vi "main.vi"() -> ()   [LabVIEW 2023] (continued)
  00000004    8        68\t00\t97\tCC\t00\t16\t39\tB4\r\n      3082  1FFFFFFF   00000004    8        00\t20\tFF\tFF\tFF\tFF\tFF\tFF\r\n      3072  1FFFFFFF   00000004    8        00\t20\tFF\tFF\tFF\tFF\tFF\tFF\r\n      3123  0CF101A7   00000004    8        68\t00\t97\tCC\t00\t16\t39\tB6\r\n      3122  1FFFFFFF   00000004    8        00\t00\tFF\tFF\tFF\tFF\tFF\tFF\r\n      3112  1FFFFFFF   00000004    8        00\t20\tFF\tFF\tFF\tFF\tFF\tFF\r\n      3103  0CF102A7   00000004    8        30\t75\tE0\t2E\t80\tFF\tFF\tFD\r\n      3103  0CF101A7   00000004    8        68\t00\t97\tCC\t00\t16\t39\tB5\r\n      3102  1FFFFFFF   00000004    8        00\t00\tFF\tFF\tFF\tFF\tFF\tFF\r\n      3093  18F106A7   00000004    8        00\tF7\tFF\tFF\tFF\tFF\tFF\tAE\r\n      3092  1FFFFFFF   00000004    8        00\t20\tFF\tFF\tFF\tFF\tFF\tFF\r\n      3083  0CF102A7   00000004    8        30\t75\tE0\t2E\t80\tFF\tFF\tFD\r\n      3083  0CF101A7   00000004    8        68\t00\t97\tCC\t00\t16\t39\tB4\r\n      3082  1FFFFFFF   00000004    8        00\t20\tFF\tFF\tFF\tFF\tFF\tFF\r\n      3123  0CF102A7   00000004    8        30\t75\tE0\t2E\t80\tFF\tFF\tFD\r\n      3123  0CF101A7   00000004    8        68\t00\t97\tCC\t00\t16\t39\tB6\r\n      3122  1FFFFFFF   00000004    8        00\t00\tFF\tFF\tFF\tFF\tFF\tFF\r\n      3112  1FFFFFFF   00000004    8        00\t20\tFF\tFF\tFF\tFF\tFF\tFF\r\n      3103  0CF102A7   00000004    8        30\t75\tE0\t2E\t80\tFF\tFF\tFD\r\n      3103  0CF101A7   00000004    8        68\t00\t97\tCC\t00\t16\t39\tB5\r\n      3102  1FFFFFFF   00000004    8        00\t00\tFF\tFF\tFF\tFF\tFF\tFF\r\n      3093  18F106A7   00000004    8        00\tF7\tFF\tFF\tFF\tFF\tFF\tAE\r\n      3092  1FFFFFFF   00000004    8        00\t20\tFF\tFF\tFF\tFF\tFF\tFF\r\n      3083  0CF102A7   00000004    8        30\t75\tE0\t2E\t80\tFF\tFF\tFD\r\n      3083  0CF101A7   00000004    8        68\t00\t97\tCC\t00\t16\t39\tB4\r\n      3132  1FFFFFFF   00000004    8        00\t20\tFF\tFF\tFF\tFF\tFF\tFF\r\n      3123  0CF102A7   00000004    8        30\t75\tE0\t2E\t80\tFF\tFF\tFD\r\n      3123  0CF101A7   00000004    8        68\t00\t97\tCC\t00\t16\t39\tB6\r\n      3122  1FFFFFFF   00000004    8        00\t00\tFF\tFF\tFF\tFF\tFF\tFF\r\n      3112  1FFFFFFF   00000004    8        00\t20\tFF\tFF\tFF\tFF\tFF\tFF\r\n      3103  0CF102A7   00000004    8        30\t75\tE0\t2E\t80\tFF\tFF\tFD\r\n      3103  0CF101A7   00000004    8        68\t00\t97\tCC\t00\t16\t39\tB5\r\n      3102  1FFFFFFF   00000004    8        00\t00\tFF\tFF\tFF\tFF\tFF\tFF\r\n      3093  18F106A7   00000004    8        00\tF7\tFF\tFF\tFF\tFF\tFF\tAE\r\n      3092  1FFFFFFF   00000004    8        00\t20\tFF\tFF\tFF\tFF\tFF\tFF\r\n      3083  0CF102A7   00000004    8        30\t75\tE0\t2E\t80\tFF\tFF\tFD\r\n      3141  18F11FF0   00000004    8        FF\t3F\t90\t68\t88\t1B\t10\t7C\r\n      3132  1FFFFFFF   00000004    8        00\t20\tFF\tFF\tFF\tFF\tFF\tFF\r\n      3123  0CF102A7   00000004    8        30\t75\tE0\t2E\t80\tFF\tFF\tFD\r\n      3123  0CF101A7   00000004    8        68\t00\t97\tCC\t00\t16\t39\tB6\r\n      3122  1FFFFFFF   00000004    8        00\t00\tFF\tFF\tFF\tFF\tFF\tFF\r\n      3112  1FFFFFFF   00000004    8        00\t20\tFF\tFF\tFF\tFF\tFF\tFF\r\n      3103  0CF102A7   00000004    8        30\t75\tE0\t2E\t80\tFF\tFF\tFD\r\n      3103  0CF101A7   00000004    8        68\t00\t97\tCC\t00\t16\t39\tB5\r\n      3102  1FFFFFFF   00000004    8        00\t00\tFF\tFF\tFF\tFF\tFF\tFF\r\n      3093  18F106A7   00000004    8        00\tF7\tFF\tFF\tFF\tFF\tFF\tAE\r\n      3092  1FFFFFFF   00000004    8        00\t20\tFF\tFF\tFF\tFF\tFF\tFF\r\n      3142  18F120F0   00000004    8        2B\t75\t60\tB1\tB0\t01\tFF\tFF\r\n      3141  18F11FF0   00000004    8        FF\t3F\t90\t68\t88\t1B\t10\t7C\r\n      3132  1FFFFFFF   00000004    8        00\t20\tFF\tFF\tFF\tFF\tFF\tFF\r\n      3123  0CF102A7   00000004    8        30\t75\tE0\t2E\t80\tFF\tFF\tFD\r\n      3123  0CF101A7   00000004    8        68\t00\t97\tCC\t00\t16\t39\tB6\r\n      3122  1FFFFFFF   00000004    8        00\t00\tFF\tFF\tFF\tFF\tFF\tFF\r\n      3112  1FFFFFFF   00000004    8        00\t20\tFF\tFF\tFF\tFF\tFF\tFF\r\n      3103  0CF102A7   00000004    8        30\t75\tE0\t2E\t80\tFF\tFF\tFD\r\n      3103  0CF101A7   00000004    8        68\t00\t97\tCC\t00\t16\t39\tB5\r\n      3102  1FFFFFFF   00000004    8        00\t00\tFF\tFF\tFF\tFF\tFF\tFF\r\n      3093  18F106A7   00000004    8        00\tF7\tFF\tFF\tFF\tFF\tFF\tAE\r\n      3143  0CF101A7   00000004    8        68\t00\t97\tCC\t00\t16\t39\tB7\r\n      3142  18F120F0   00000004    8        2B\t75\t60\tB1\tB0\t01\tFF\tFF\r\n      3141  18F11FF0   00000004    8        FF\t3F\t90\t68\t88\t1B\t10\t7C\r\n      3132  1FFFFFFF   00000004    8        00\t20\tFF\tFF\tFF\tFF\tFF\tFF\r\n      3123  0CF102A7   00000004    8        30\t75\tE0\t2E\t80\tFF\tFF\tFD\r\n      3123  0CF101A7   00000004    8        68\t00\t97\tCC\t00\t16\t39\tB6\r\n      3122  1FFFFFFF   00000004    8        00\t00\tFF\tFF\tFF\tFF\tFF\tFF\r\n      3112  1FFFFFFF   00000004    8        00\t20\tFF\tFF\tFF\tFF\tFF\tFF\r\n      3103  0CF102A7   00000004    8        30\t75\tE0\t2E\t80\tFF\tFF\tFD\r\n      3103  0CF101A7   00000004    8        68\t00\t97\tCC\t00\t16\t39\tB5\r\n      3102  1FFFFFFF   00000004    8        00\t00\tFF\tFF\tFF\tFF\tFF\tFF\r\n      3143  0CF102A7   00000004    8        30\t75\tE0\t2E\t80\tFF\tFF\tFD\r\n      3143  0CF101A7   00000004    8        68\t00\t97\tCC\t00\t16\t39\tB7\r\n      3142  18F120F0   00000004    8        2B\t75\t60\tB1\tB0\t01\tFF\tFF\r\n      3141  18F11FF0   00000004    8        FF\t3F\t90\t68\t88\t1B\t10\t7C\r\n      3132  1FFFFFFF   00000004    8        00\t20\tFF\tFF\tFF\tFF\tFF\tFF\r\n      3123  0CF102A7   00000004    8        30\t75\tE0\t2E\t80\tFF\tFF\tFD\r\n      3123  0CF101A7   00000004    8        68\t00\t97\tCC\t00\t16\t39\tB6\r\n      3122  1FFFFFFF   00000004    8        00\t00\tFF\tFF\tFF\tFF\tFF\tFF\r\n      3112  1FFFFFFF   00000004    8        00\t20\tFF\tFF\tFF\tFF\tFF\tFF\r\n      3103  0CF102A7   00000004    8        30\t75\tE0\t2E\t80\tFF\tFF\tFD\r\n      3103  0CF101A7   00000004    8        68\t00\t97\tCC\t00\t16\t39\tB5\r\n      3144  0C3C4D4A   00000004    8        BE\tFF\tFF\t7F\t18\tFF\tFF\t57\r\n      3143  0CF102A7   00000004    8        30\t75\tE0\t2E\t80\tFF\tFF\tFD\r\n      3143  0CF101A7   00000004    8        68\t00\t97\tCC\t00\t16\t39\tB7\r\n      3142  18F120F0   00000004    8        2B\t75\t60\tB1\tB0\t01\tFF\tFF\r\n      3141  18F11FF0   00000004    8        FF\t3F\t90\t68\t88\t1B\t10\t7C\r\n      3132  1FFFFFFF   00000004    8        00\t20\tFF\tFF\tFF\tFF\tFF\tFF\r\n      3123  0CF102A7   00000004    8        30\t75\tE0\t2E\t80\tFF\tFF\tFD\r\n      3123  0CF101A7   00000004    8        68\t00\t97\tCC\t00\t16\t39\tB6\r\n      3122  1FFFFFFF   00000004    8        00\t00\tFF\tFF\tFF\tFF\tFF\tFF\r\n      3112  1FFFFFFF   00000004    8        00\t20\tFF\tFF\tFF\tFF\tFF\tFF\r\n      3103  0CF102A7   00000004    8        30\t75\tE0\t2E\t80\tFF\tFF\tFD\r\n      3144  0CF103A7   00000004    8        17\t1F\t08\t60\tB1\t1F\t08\t57\r\n      3144  0C3C4D4A   00000004    8        BE\tFF\tFF\t7F\t18\tFF\tFF\t57\r\n      3143  0CF102A7   00000004    8        30\t75\tE0\t2E\t80\tFF\tFF\tFD\r\n      3143  0CF101A7   00000004    8        68\t00\t97\tCC\t00\t16\t39\tB7\r\n      3142  18F120F0   00000004    8        2B\t75\t60\tB1\tB0\t01\tFF\tFF\r\n      3141  18F11FF0   00000004    8        FF\t3F\t90\t68\t88\t1B\t10\t7C\r\n      3132  1FFFFFFF   00000004    8        00\t20\tFF\tFF\tFF\tFF\tFF\tFF\r\n      3123  0CF102A7   00000004    8        30\t75\tE0\t2E\t80\tFF\tFF\tFD\r\n      3123  0CF101A7   00000004    8        68\t00\t97\tCC\t00\t16\t39\tB6\r\n      3122  1FFFFFFF   00000004    8        00\t00\tFF\tFF\tFF\tFF\tFF\tFF\r\n      3112  1FFFFFFF   00000004    8        00\t20\tFF\tFF\tFF\tFF\tFF\tFF\r\n      3145  0CF104A7   00000004    8        F0\t60\t22\tFC\tFF\tFF\tFF\t57\r\n      3144  0CF103A7   00000004    8        17\t1F\t08\t60\tB1\t1F\t08\t57\r\n      3144  0C3C4D4A   00000004    8        BE\tFF\tFF\t7F\t18\tFF\tFF\t57\r\n      3143  0CF102A7   00000004    8        30\t75\tE0\t2E\t80\tFF\tFF\tFD\r\n      3143  0CF101A7   00000004    8        68\t00\t97\tCC\t00\t16\t39\tB7\r\n      3142  18F120F0   00000004    8        2B\t75\t60\tB1\tB0\t01\tFF\tFF\r\n      3141  18F11FF0   00000004    8        FF\t3F\t90\t68\t88\t1B\t10\t7C\r\n      3132  1FFFFFFF   00000004    8        00\t20\tFF\tFF\tFF\tFF\tFF\tFF\r\n      3123  0CF102A7   00000004    8        30\t75\tE0\t2E\t80\tFF\tFF\tFD\r\n      3123  0CF101A7   00000004    8        68\t00\t97\tCC\t00\t16\t39\tB6\r\n      3122  1FFFFFFF   00000004    8        00\t00\tFF\tFF\tFF\tFF\tFF\tFF\r\n      3145  18F106A7   00000004    8        00\tF7\tFF\tFF\tFF\tFF\tFF\tAF\r\n      3145  0CF104A7   00000004    8        F0\t60\t22\tFC\tFF\tFF\tFF\t57\r\n      3144  0CF103A7   00000004    8        17\t1F\t08\t60\tB1\t1F\t08\t57\r\n      3144  0C3C4D4A   00000004    8        BE\tFF\tFF\t7F\t18\tFF\tFF\t57\r\n      3143  0CF102A7   00000004    8        30\t75\tE0\t2E\t80\tFF\tFF\tFD\r\n      3143  0CF101A7   00000004    8        68\t00\t97\tCC\t00\t16\t39\tB7\r\n      3142  18F120F0   00000004    8        2B\t75\t60\tB1\tB0\t01\tFF\tFF\r\n      3141  18F11FF0   00000004    8        FF\t3F\t90\t68\t88\t1B\t10\t7C\r\n      3132  1FFFFFFF   00000004    8        00\t20\tFF\tFF\tFF\tFF\tFF\tFF\r\n      3123  0CF102A7   00000004    8        30\t75\tE0\t2E\t80\tFF\tFF\tFD\r\n      3123  0CF101A7   00000004    8        68\t00\t97\tCC\t00\t16\t39\tB6\r\n      3146  18F108A7   00000004    8        F0\t00\t00\tFF\tFF\tFF\tFF\t44\r\n      3145  18F106A7   00000004    8        00\tF7\tFF\tFF\tFF\tFF\tFF\tAF\r\n      3145  0CF104A7   00000004    8        F0\t60\t22\tFC\tFF\tFF\tFF\t57\r\n      3144  0CF103A7   00000004    8        17\t1F\t08\t60\tB1\t1F\t08\t57\r\n      3144  0C3C4D4A   00000004    8        BE\tFF\tFF\t7F\t18\tFF\tFF\t57\r\n      3143  0CF102A7   00000004    8        30\t75\tE0\t2E\t80\tFF\tFF\tFD\r\n      3143  0CF101A7   00000004    8        68\t00\t97\tCC\t00\t16\t39\tB7\r\n      3142  18F120F0   00000004    8        2B\t75\t60\tB1\tB0\t01\tFF\tFF\r\n      3141  18F11FF0   00000004    8        FF\t3F\t90\t68\t88\t1B\t10\t7C\r\n      3132  1FFFFFFF   00000004    8        00\t20\tFF\tFF\tFF\tFF\tFF\tFF\r\n      3123  0CF102A7   00000004    8        30\t75\tE0\t2E\t80\tFF\tFF\tFD\r\n      3146  18F121F0   00000004    8        09\t33\t00\t00\tFF\tFF\tB0\t01\r\n      3146  18F108A7   00000004    8        F0\t00\t00\tFF\tFF\tFF\tFF\t44\r\n      3145  18F106A7   00000004    8        00\tF7\tFF\tFF\tFF\tFF\tFF\tAF\r\n      3145  0CF104A7   00000004    8        F0\t60\t22\tFC\tFF\tFF\tFF\t57\r\n      3144  0CF103A7   00000004    8        17\t1F\t08\t60\tB1\t1F\t08\t57\r\n      3144  0C3C4D4A   00000004    8        BE\tFF\tFF\t7F\t18\tFF\tFF\t57\r\n      3143  0CF102A7   00000004    8        30\t75\tE0\t2E\t80\tFF\tFF\tFD\r\n      3143  0CF101A7   00000004    8        68\t00\t97\tCC\t00\t16\t39\tB7\r\n      3142  18F120F0   00000004    8        2B\t75\t60\tB1\tB0\t01\tFF\tFF\r\n      3141  18F11FF0   00000004    8        FF\t3F\t90\t68\t88\t1B\t10\t7C\r\n      3132  1FFFFFFF   00000004    8        00\t20\tFF\tFF\tFF\tFF\tFF\tFF\r\n      3147  18FEF117   00000004    8        F7\t97\tCC\tCF\tFF\tFF\tFF\tFF\r\n      3146  18F121F0   00000004    8        09\t33\t00\t00\tFF\tFF\tB0\t01\r\n      3146  18F108A7   00000004    8        F0\t00\t00\tFF\tFF\tFF\tFF\t44\r\n      3145  18F106A7   00000004    8        00\tF7\tFF\tFF\tFF\tFF\tFF\tAF\r\n      3145  0CF104A7   00000004    8        F0\t60\t22\tFC\tFF\tFF\tFF\t57\r\n      3144  0CF103A7   00000004    8        17\t1F\t08\t60\tB1\t1F\t08\t57\r\n      3144  0C3C4D4A   00000004    8        BE\tFF\tFF\t7F\t18\tFF\tFF\t57\r\n      3143  0CF102A7   00000004    8        30\t75\tE0\t2E\t80\tFF\tFF\tFD\r\n      3143  0CF101A7   00000004    8        68\t00\t97\tCC\t00\t16\t39\tB7\r\n      3142  18F120F0   00000004    8        2B\t75\t60\tB1\tB0\t01\tFF\tFF\r\n      3141  18F11FF0   00000004    8        FF\t3F\t90\t68\t88\t1B\t10\t7C\r\n      3148  1FFFFFFF   00000004    8        00\t00\tFF\tFF\tFF\tFF\tFF\tFF\r\n      3147  18FEF117   00000004    8        F7\t97\tCC\tCF\tFF\tFF\tFF\tFF\r\n      3146  18F121F0   00000004    8        09\t33\t00\t00\tFF\tFF\tB0\t01\r\n      3146  18F108A7   00000004    8        F0\t00\t00\tFF\tFF\tFF\tFF\t44\r\n      3145  18F106A7   00000004    8        00\tF7\tFF\tFF\tFF\tFF\tFF\tAF\r\n      3145  0CF104A7   00000004    8        F0\t60\t22\tFC\tFF\tFF\tFF\t57\r\n      3144  0CF103A7   00000004    8        17\t1F\t08\t60\tB1\t1F\t08\t57\r\n      3144  0C3C4D4A   00000004    8        BE\tFF\tFF\t7F\t18\tFF\tFF\t57\r\n      3143  0CF102A7   00000004    8        30\t75\tE0\t2E\t80\tFF\tFF\tFD\r\n      3143  0CF101A7   00000004    8        68\t00\t97\tCC\t00\t16\t39\tB7\r\n      3142  18F120F0   00000004    8        2B\t75\t60\tB1\tB0\t01\tFF\tFF\r\n      3152  1FFFFFFF   00000004    8        00\t00\tFF\tFF\tFF\tFF\tFF\tFF\r\n      3148  1FFFFFFF   00000004    8        00\t00\tFF\tFF\tFF\tFF\tFF\tFF\r\n      3147  18FEF117   00000004    8        F7\t97\tCC\tCF\tFF\tFF\tFF\tFF\r\n      3146  18F121F0   00000004    8        09\t33\t00\t00\tFF\tFF\tB0\t01\r\n      3146  18F108A7   00000004    8        F0\t00\t00\tFF\tFF\tFF\tFF\t44\r\n      3145  18F106A7   00000004    8        00\tF7\tFF\tFF\tFF\tFF\tFF\tAF\r\n      3145  0CF104A7   00000004    8        F0\t60\t22\tFC\tFF\tFF\tFF\t57\r\n      3144  0CF103A7   00000004    8        17\t1F\t08\t60\tB1\t1F\t08\t57\r\n      3144  0C3C4D4A   00000004    8        BE\tFF\tFF\t7F\t18\tFF\tFF\t57\r\n      3143  0CF102A7   00000004    8        30\t75\tE0\t2E\t80\tFF\tFF\tFD\r\n      3143  0CF101A7   00000004    8        68\t00\t97\tCC\t00\t16\t39\tB7\r\n      3162  1FFFFFFF   00000004    8        00\t00\tFF\tFF\tFF\tFF\tFF\tFF\r\n      3152  1FFFFFFF   00000004    8        00\t00\tFF\tFF\tFF\tFF\tFF\tFF\r\n      3148  1FFFFFFF   00000004    8        00\t00\tFF\tFF\tFF\tFF\tFF\tFF\r\n      3147  18FEF117   00000004    8        F7\t97\tCC\tCF\tFF\tFF\tFF\tFF\r\n      3146  18F121F0   00000004    8        09\t33\t00\t00\tFF\tFF\tB0\t01\r\n      3146  18F108A7   00000004    8        F0\t00\t00\tFF\tFF\tFF\tFF\t44\r\n      3145  18F106A7   00000004    8        00\tF7\tFF\tFF\tFF\tFF\tFF\tAF\r\n      3145  0CF104A7   00000004    8        F0\t60\t22\tFC\tFF\tFF\tFF\t57\r\n      3144  0CF103A7   00000004    8        17\t1F\t08\t60\tB1\t1F\t08\t57\r\n      3144  0C3C4D4A   00000004    8        BE\tFF\tFF\t7F\t18\tFF\tFF\t57\r\n      3143  0CF102A7   00000004    8        30\t75\tE0\t2E\t80\tFF\tFF\tFD\r\n      3163  0CF101A7   00000004    8        68\t00\t97\tCC\t00\t16\t39\tB8\r\n      3162  1FFFFFFF   00000004    8        00\t00\tFF\tFF\tFF\tFF\tFF\tFF\r\n      3152  1FFFFFFF   00000004    8        00\t00\tFF\tFF\tFF\tFF\tFF\tFF\r\n      3148  1FFFFFFF   00000004    8        00\t00\tFF\tFF\tFF\tFF\tFF\tFF\r\n      3147  18FEF117   00000004    8        F7\t97\tCC\tCF\tFF\tFF\tFF\tFF\r\n      3146  18F121F0   00000004    8        09\t33\t00\t00\tFF\tFF\tB0\t01\r\n      3146  18F108A7   00000004    8        F0\t00\t00\tFF\tFF\tFF\tFF\t44\r\n      3145  18F106A7   00000004    8        00\tF7\tFF\tFF\tFF\tFF\tFF\tAF\r\n      3145  0CF104A7   00000004    8        F0\t60\t22\tFC\tFF\tFF\tFF\t57\r\n      3144  0CF103A7   00000004    8        17\t1F\t08\t60\tB1\t1F\t08\t57\r\n      3144  0C3C4D4A   00000004    8        BE\tFF\tFF\t7F\t18\tFF\tFF\t57\r\n      3163  0CF102A7   00000004    8        30\t75\tE0\t2E\t80\tFF\tFF\tFD\r\n      3163  0CF101A7   00000004    8        68\t00\t97\tCC\t00\t16\t39\tB8\r\n      3162  1FFFFFFF   00000004    8        00\t00\tFF\tFF\tFF\tFF\tFF\tFF\r\n      3152  1FFFFFFF   00000004    8        00\t00\tFF\tFF\tFF\tFF\tFF\tFF\r\n      3148  1FFFFFFF   00000004    8        00\t00\tFF\tFF\tFF\tFF\tFF\tFF\r\n      3147  18FEF117   00000004    8        F7\t97\tCC\tCF\tFF\tFF\tFF\tFF\r\n      3146  18F121F0   00000004    8        09\t33\t00\t00\tFF\tFF\tB0\t01\r\n      3146  18F108A7   00000004    8        F0\t00\t00\tFF\tFF\tFF\tFF\t44\r\n      3145  18F106A7   00000004    8        00\tF7\tFF\tFF\tFF\tFF\tFF\tAF\r\n      3145  0CF104A7   00000004    8        F0\t60\t22\tFC\tFF\tFF\tFF\t57\r\n      3144  0CF103A7   00000004    8        17\t1F\t08\t60\tB1\t1F\t08\t57\r\n      3172  1FFFFFFF   00000004    8        00\t00\tFF\tFF\tFF\tFF\tFF\tFF\r\n      3163  0CF102A7   00000004    8        30\t75\tE0\t2E\t80\tFF\tFF\tFD\r\n      3163  0CF101A7   00000004    8        68\t00\t97\tCC\t00\t16\t39\tB8\r\n      3162  1FFFFFFF   00000004    8        00\t00\tFF\tFF\tFF\tFF\tFF\tFF\r\n      3152  1FFFFFFF   00000004    8        00\t00\tFF\tFF\tFF\tFF\tFF\tFF\r\n      3148  1FFFFFFF   00000004    8        00\t00\tFF\tFF\tFF\tFF\tFF\tFF\r\n      3147  18FEF117   00000004    8        F7\t97\tCC\tCF\tFF\tFF\tFF\tFF\r\n      3146  18F121F0   00000004    8        09\t33\t00\t00\tFF\tFF\tB0\t01\r\n      3146  18F108A7   00000004    8        F0\t00\t00\tFF\tFF\tFF\tFF\t44\r\n      3145  18F106A7   00000004    8        00\tF7\tFF\tFF\tFF\tFF\tFF\tAF\r\n      3145  0CF104A7   00000004    8        F0\t60\t22\tFC\tFF\tFF\tFF\t57\r\n      3182  1FFFFFFF   00000004    8        00\t00\tFF\tFF\tFF\tFF\tFF\tFF\r\n      3172  1FFFFFFF   00000004    8        00\t00\tFF\tFF\tFF\tFF\tFF\tFF\r\n      3163  0CF102A7   00000004    8        30\t75\tE0\t2E\t80\tFF\tFF\tFD\r\n      3163  0CF101A7   00000004    8        68\t00\t97\tCC\t00\t16\t39\tB8\r\n      3162  1FFFFFFF   00000004    8        00\t00\tFF\tFF\tFF\tFF\tFF\tFF\r\n      3152  1FFFFFFF   00000004    8        00\t00\tFF\tFF\tFF\tFF\tFF\tFF\r\n      3148  1FFFFFFF   00000004    8        00\t00\tFF\tFF\tFF\tFF\tFF\tFF\r\n      3147  18FEF117   00000004    8        F7\t97\tCC\tCF\tFF\tFF\tFF\tFF\r\n      3146  18F121F0   00000004    8        09\t33\t00\t00\tFF\tFF\tB0\t01\r\n      3146  18F108A7   00000004    8        F0\t00\t00\tFF\tFF\tFF\tFF\t44\r\n      3145  18F106A7   00000004    8        00\tF7\tFF\tFF\tFF\tFF\tFF\tAF\r\n      3183  0CF101A7   00000004    8        68\t00\t97\tCC\t00\t16\t39\tB9\r\n      3182  1FFFFFFF   00000004    8        00\t00\tFF\tFF\tFF\tFF\tFF\tFF\r\n      3172  1FFFFFFF   00000004    8        00\t00\tFF\tFF\tFF\tFF\tFF\tFF\r\n      3163  0CF102A7   00000004    8        30\t75\tE0\t2E\t80\tFF\tFF\tFD\r\n      3163  0CF101A7   00000004    8        68\t00\t97\tCC\t00\t16\t39\tB8\r\n      3162  1FFFFFFF   00000004    8        00\t00\tFF\tFF\tFF\tFF\tFF\tFF\r\n      3152  1FFFFFFF   00000004    8        00\t00\tFF\tFF\tFF\tFF\tFF\tFF\r\n      3148  1FFFFFFF   00000004    8        00\t00\tFF\tFF\tFF\tFF\tFF\tFF\r\n      3147  18FEF117   00000004    8        F7\t97\tCC\tCF\tFF\tFF\tFF\tFF\r\n      3146  18F121F0   00000004    8        09\t33\t00\t00\tFF\tFF\tB0\t01\r\n      3146  18F108A7   00000004    8        F0\t00\t00\tFF\tFF\tFF\tFF\t44\r\n      3183  0CF102A7   00000004    8        30\t75\tE0\t2E\t80\tFF\tFF\tFD\r\n      3183  0CF101A7   00000004    8        68\t00\t97\tCC\t00\t16\t39\tB9\r\n      3182  1FFFFFFF   00000004    8        00\t00\tFF\tFF\tFF\tFF\tFF\tFF\r\n      3172  1FFFFFFF   00000004    8        00\t00\tFF\tFF\tFF\tFF\tFF\tFF\r\n      3163  0CF102A7   00000004    8        30\t75\tE0\t2E\t80\tFF\tFF\tFD\r\n      3163  0CF101A7   00000004    8        68\t00\t97\tCC\t00\t16\t39\tB8\r\n      3162  1FFFFFFF   00000004    8        00\t00\tFF\tFF\tFF\tFF\tFF\tFF\r\n      3152  1FFFFFFF   00000004    8        00\t00\tFF\tFF\tFF\tFF\tFF\tFF\r\n      3148  1FFFFFFF   00000004    8        00\t00\tFF\tFF\tFF\tFF\tFF\tFF\r\n      3147  18FEF117   00000004    8        F7\t97\tCC\tCF\tFF\tFF\tFF\tFF\r\n      3146  18F121F0   00000004    8        09\t33\t00\t00\tFF\tFF\tB0\t01\r\n      3192  1FFFFFFF   00000004    8        00\t00\tFF\tFF\tFF\tFF\tFF\tFF\r\n      3183  0CF102A7   00000004    8        30\t75\tE0\t2E\t80\tFF\tFF\tFD\r\n      3183  0CF101A7   00000004    8        68\t00\t97\tCC\t00\t16\t39\tB9\r\n      3182  1FFFFFFF   00000004    8        00\t00\tFF\tFF\tFF\tFF\tFF\tFF\r\n      3172  1FFFFFFF   00000004    8        00\t00\tFF\tFF\tFF\tFF\tFF\tFF\r\n      3163  0CF102A7   00000004    8        30\t75\tE0\t2E\t80\tFF\tFF\tFD\r\n      3163  0CF101A7   00000004    8        68\t00\t97\tCC\t00\t16\t39\tB8\r\n      3162  1FFFFFFF   00000004    8        00\t00\tFF\tFF\tFF\tFF\tFF\tFF\r\n      3152  1FFFFFFF   00000004    8        00\t00\tFF\tFF\tFF\tFF\tFF\tFF\r\n      3148  1FFFFFFF   00000004    8        00\t00\tFF\tFF\tFF\tFF\tFF\tFF\r\n      3147  18FEF117   00000004    8        F7\t97\tCC\tCF\tFF\tFF\tFF\tFF\r\n      3193  18F106A7   00000004    8        00\tF7\tFF\tFF\tFF\tFF\tFF\tB0\r\n      3192  1FFFFFFF   00000004    8        00\t00\tFF\tFF\tFF\tFF\tFF\tFF\r\n      3183  0CF102A7   00000004    8        30\t75\tE0\t2E\t80\tFF\tFF\tFD\r\n      3183  0CF101A7   00000004    8        68\t00\t97\tCC\t00\t16\t39\tB9\r\n      3182  1FFFFFFF   00000004    8        00\t00\tFF\tFF\tFF\tFF\tFF\tFF\r\n      3172  1FFFFFFF   00000004    8        00\t00\tFF\tFF\tFF\tFF\tFF\tFF\r\n      3163  0CF102A7   00000004    8        30\t75\tE0\t2E\t80\tFF\tFF\tFD\r\n      3163  0CF101A7   00000004    8        68\t00\t97\tCC\t00\t16\t39\tB8\r\n      3162  1FFFFFFF   00000004    8        00\t00\tFF\tFF\tFF\tFF\tFF\tFF\r\n      3152  1FFFFFFF   00000004    8        00\t00\tFF\tFF\tFF\tFF\tFF\tFF\r\n      3148  1FFFFFFF   00000004    8        00\t00\tFF\tFF\tFF\tFF\tFF\tFF\r\n      3202  1FFFFFFF   00000004    8        00\t00\tFF\tFF\tFF\tFF\tFF\tFF\r\n      3193  18F106A7   00000004    8        00\tF7\tFF\tFF\tFF\tFF\tFF\tB0\r\n      3192  1FFFFFFF   00000004    8        00\t00\tFF\tFF\tFF\tFF\tFF\tFF\r\n      3183  0CF102A7   00000004    8        30\t75\tE0\t2E\t80\tFF\tFF\tFD\r\n      3183  0CF101A7   00000004    8        68\t00\t97\tCC\t00\t16\t39\tB9\r\n      3182  1FFFFFFF   00000004    8        00\t00\tFF\tFF\tFF\tFF\tFF\tFF\r\n      3172  1FFFFFFF   00000004    8        00\t00\tFF\tFF\tFF\tFF\tFF\tFF\r\n      3163  0CF102A7   00000004    8        30\t75\tE0\t2E\t80\tFF\tFF\tFD\r\n      3163  0CF101A7   00000004    8        68\t00\t97\tCC\t00\t16\t39\tB8\r\n      3162  1FFFFFFF   00000004    8        00\t00\tFF\tFF\tFF\tFF\tFF\tFF\r\n      3152  1FFFFFFF   00000004    8        00\t00\tFF\tFF\tFF\tFF\tFF\tFF\r\n      3203  0CF101A7   00000004    8        68\t00\t97\tCC\t00\t16\t39\tBA\r\n      3202  1FFFFFFF   00000004    8        00\t00\tFF\tFF\tFF\tFF\tFF\tFF\r\n      3193  18F106A7   00000004    8        00\tF7\tFF\tFF\tFF\tFF\tFF\tB0\r\n      3192  1FFFFFFF   00000004    8        00\t00\tFF\tFF\tFF\tFF\tFF\tFF\r\n      3183  0CF102A7   00000004    8        30\t75\tE0\t2E\t80\tFF\tFF\tFD\r\n      3183  0CF101A7   00000004    8        68\t00\t97\tCC\t00\t16\t39\tB9\r\n      3182  1FFFFFFF   00000004    8        00\t00\tFF\tFF\tFF\tFF\tFF\tFF\r\n      3172  1FFFFFFF   00000004    8        00\t00\tFF\tFF\tFF\tFF\tFF\tFF\r\n      3163  0CF102A7   00000004    8        30\t75\tE0\t2E\t80\tFF\tFF\tFD\r\n      3163  0CF101A7   00000004    8        68\t00\t97\tCC\t00\t16\t39\tB8\r\n      3162  1FFFFFFF   00000004    8        00\t00\tFF\tFF\tFF\tFF\tFF\tFF\r\n      3203  0CF102A7   00000004    8        30\t75\tE0\t2E\t80\tFF\tFF\tFD\r\n      3203  0CF101A7   00000004    8        68\t00\t97\tCC\t00\t16\t39\tBA\r\n      3202  1FFFFFFF   00000004    8        00\t00\tFF\tFF\tFF\tFF\tFF\tFF\r\n      3193  18F106A7   00000004    8        00\tF7\tFF\tFF\tFF\tFF\tFF\tB0\r\n      3192  1FFFFFFF   00000004    8        00\t00\tFF\tFF\tFF\tFF\tFF\tFF\r\n      3183  0CF102A7   00000004    8        30\t75\tE0\t2E\t80\tFF\tFF\tFD\r\n      3183  0CF101A7   00000004    8        68\t00\t97\tCC\t00\t16\t39\tB9\r\n      3182  1FFFFFFF   00000004    8        00\t00\tFF\tFF\tFF\tFF\tFF\tFF\r\n      3172  1FFFFFFF   00000004    8        00\t00\tFF\tFF\tFF\tFF\tFF\tFF\r\n      3163  0CF102A7   00000004    8        30\t75\tE0\t2E\t80\tFF\tFF\tFD\r\n      3163  0CF101A7   00000004    8        68\t00\t97\tCC\t00\t16\t39\tB8\r\n      3212  1FFFFFFF   00000004    8        00\t00\tFF\tFF\tFF\tFF\tFF\tFF\r\n      3203  0CF102A7   00000004    8        30\t75\tE0\t2E\t80\tFF\tFF\tFD\r\n      3203  0CF101A7   00000004    8        68\t00\t97\tCC\t00\t16\t39\tBA\r\n      3202  1FFFFFFF   00000004    8        00\t00\tFF\tFF\tFF\tFF\tFF\tFF\r\n      3193  18F106A7   00000004    8        00\tF7\tFF\tFF\tFF\tFF\tFF\tB0\r\n      3192  1FFFFFFF   00000004    8        00\t00\tFF\tFF\tFF\tFF\tFF\tFF\r\n      3183  0CF102A7   00000004    8        30\t75\tE0\t2E\t80\tFF\tFF\tFD\r\n      3183  0CF101A7   00000004    8        68\t00\t97\tCC\t00\t16\t39\tB9\r\n      3182  1FFFFFFF   00000004    8        00\t00\tFF\tFF\tFF\tFF\tFF\tFF\r\n      3172  1FFFFFFF   00000004    8        00\t00\tFF\tFF\tFF\tFF\tFF\tFF\r\n      3163  0CF102A7   00000004    8        30\t75\tE0\t2E\t80\tFF\tFF\tFD\r\n      3222  1FFFFFFF   00000004    8        00\t20\tFF\tFF\tFF\tFF\tFF\tFF\r\n      3212  1FFFFFFF   00000004    8        00\t00\tFF\tFF\tFF\tFF\tFF\tFF\r\n      3203  0CF102A7   00000004    8        30\t75\tE0\t2E\t80\tFF\tFF\tFD\r\n      3203  0CF101A7   00000004    8        68\t00\t97\tCC\t00\t16\t39\tBA\r\n      3202  1FFFFFFF   00000004    8        00\t00\tFF\tFF\tFF\tFF\tFF\tFF\r\n      3193  18F106A7   00000004    8        00\tF7\tFF\tFF\tFF\tFF\tFF\tB0\r\n      3192  1FFFFFFF   00000004    8        00\t00\tFF\tFF\tFF\tFF\tFF\tFF\r\n      3183  0CF102A7   00000004    8        30\t75\tE0\t2E\t80\tFF\tFF\tFD\r\n      3183  0CF101A7   00000004    8        68\t00\t97\tCC\t00\t16\t39\tB9\r\n      3182  1FFFFFFF   00000004    8        00\t00\tFF\tFF\tFF\tFF\tFF\tFF\r\n      3172  1FFFFFFF   00000004    8        00\t00\tFF\tFF\tFF\tFF\tFF\tFF\r\n      3223  0CF101A7   00000004    8        68\t00\t97\tCC\t00\t00\t39\tBB\r\n      3222  1FFFFFFF   00000004    8        00\t20\tFF\tFF\tFF\tFF\tFF\tFF\r\n      3212  1FFFFFFF   00000004    8        00\t00\tFF\tFF\tFF\tFF\tFF\tFF\r\n      3203  0CF102A7   00000004    8        30\t75\tE0\t2E\t80\tFF\tFF\tFD\r\n      3203  0CF101A7   00000004    8        68\t00\t97\tCC\t00\t16\t39\tBA\r\n      3202  1FFFFFFF   00000004    8        00\t00\tFF\tFF\tFF\tFF\tFF\tFF\r\n      3193  18F106A7   00000004    8        00\tF7\tFF\tFF\tFF\tFF\tFF\tB0\r\n      3192  1FFFFFFF   00000004    8        00\t00\tFF\tFF\tFF\tFF\tFF\tFF\r\n      3183  0CF102A7   00000004    8        30\t75\tE0\t2E\t80\tFF\tFF\tFD\r\n      3183  0CF101A7   00000004    8        68\t00\t97\tCC\t00\t16\t39\tB9\r\n      3182  1FFFFFFF   00000004    8        00\t00\tFF\tFF\tFF\tFF\tFF\tFF\r\n      3223  0CF102A7   00000004    8        30\t75\tE0\t2E\t80\tFF\tFF\tFD\r\n      3223  0CF101A7   00000004    8        68\t00\t97\tCC\t00\t00\t39\tBB\r\n      3222  1FFFFFFF   00000004    8        00\t20\tFF\tFF\tFF\tFF\tFF\tFF\r\n      3212  1FFFFFFF   00000004    8        00\t00\tFF\tFF\tFF\tFF\tFF\tFF\r\n      3203  0CF102A7   00000004    8        30\t75\tE0\t2E\t80\tFF\tFF\tFD\r\n      3203  0CF101A7   00000004    8        68\t00\t97\tCC\t00\t16\t39\tBA\r\n      3202  1FFFFFFF   00000004    8        00\t00\tFF\tFF\tFF\tFF\tFF\tFF\r\n      3193  18F106A7   00000004    8        00\tF7\tFF\tFF\tFF\tFF\tFF\tB0\r\n      3192  1FFFFFFF   00000004    8        00\t00\tFF\tFF\tFF\tFF\tFF\tFF\r\n      3183  0CF102A7   00000004    8        30\t75\tE0\t2E\t80\tFF\tFF\tFD\r\n      3183  0CF101A7   00000004    8        68\t00\t97\tCC\t00\t16\t39\tB9\r\n      3232  1FFFFFFF   00000004    8        00\t00\tFF\tFF\tFF\tFF\tFF\tFF\r\n      3223  0CF102A7   00000004    8        30\t75\tE0\t2E\t80\tFF\tFF\tFD\r\n      3223  0CF101A7   00000004    8        68\t00\t97\tCC\t00\t00\t39\tBB\r\n      3222  1FFFFFFF   00000004    8        00\t20\tFF\tFF\tFF\tFF\tFF\tFF\r\n      3212  1FFFFFFF   00000004    8        00\t00\tFF\tFF\tFF\tFF\tFF\tFF\r\n      3203  0CF102A7   00000004    8        30\t75\tE0\t2E\t80\tFF\tFF\tFD\r\n      3203  0CF101A7   00000004    8        68\t00\t97\tCC\t00\t16\t39\tBA\r\n      3202  1FFFFFFF   00000004    8        00\t00\tFF\tFF\tFF\tFF\tFF\tFF\r\n      3193  18F106A7   00000004    8        00\tF7\tFF\tFF\tFF\tFF\tFF\tB0\r\n      3192  1FFFFFFF   00000004    8        00\t00\tFF\tFF\tFF\tFF\tFF\tFF\r\n      3183  0CF102A7   00000004    8        30\t75\tE0\t2E\t80\tFF\tFF\tFD\r\n      3241  18F11FF0   00000004    8        FF\t3F\t90\t68\t88\t1B\t10\t8C\r\n      3232  1FFFFFFF   00000004    8        00\t00\tFF\tFF\tFF\tFF\tFF\tFF\r\n      3223  0CF102A7   00000004    8        30\t75\tE0\t2E\t80\tFF\tFF\tFD\r\n      3223  0CF101A7   00000004    8        68\t00\t97\tCC\t00\t00\t39\tBB\r\n      3222  1FFFFFFF   00000004    8        00\t20\tFF\tFF\tFF\tFF\tFF\tFF\r\n      3212  1FFFFFFF   00000004    8        00\t00\tFF\tFF\tFF\tFF\tFF\tFF\r\n      3203  0CF102A7   00000004    8        30\t75\tE0\t2E\t80\tFF\tFF\tFD\r\n      3203  0CF101A7   00000004    8        68\t00\t97\tCC\t00\t16\t39\tBA\r\n      3202  1FFFFFFF   00000004    8        00\t00\tFF\tFF\tFF\tFF\tFF\tFF\r\n      3193  18F106A7   00000004    8        00\tF7\tFF\tFF\tFF\tFF\tFF\tB0\r\n      3192  1FFFFFFF   00000004    8        00\t00\tFF\tFF\tFF\tFF\tFF\tFF\r\n      3242  18F120F0   00000004    8        2B\t75\t60\tB1\tB0\t01\tFF\tFF\r\n      3241  18F11FF0   00000004    8        FF\t3F\t90\t68\t88\t1B\t10\t8C\r\n      3232  1FFFFFFF   00000004    8        00\t00\tFF\tFF\tFF\tFF\tFF\tFF\r\n      3223  0CF102A7   00000004    8        30\t75\tE0\t2E\t80\tFF\tFF\tFD\r\n      3223  0CF101A7   00000004    8        68\t00\t97\tCC\t00\t00\t39\tBB\r\n      3222  1FFFFFFF   00000004    8        00\t20\tFF\tFF\tFF\tFF\tFF\tFF\r\n      3212  1FFFFFFF   00000004    8        00\t00\tFF\tFF\tFF\tFF\tFF\tFF\r\n      3203  0CF102A7   00000004    8        30\t75\tE0\t2E\t80\tFF\tFF\tFD\r\n      3203  0CF101A7   00000004    8        68\t00\t97\tCC\t00\t16\t39\tBA\r\n      3202  1FFFFFFF   00000004    8        00\t00\tFF\tFF\tFF\tFF\tFF\tFF\r\n      3193  18F106A7   00000004    8        00\tF7\tFF\tFF\tFF\tFF\tFF\tB0\r\n      3243  0CF101A7   00000004    8        68\t00\t97\tCC\t00\t00\t39\tBC\r\n      3242  18F120F0   00000004    8        2B\t75\t60\tB1\tB0\t01\tFF\tFF\r\n      3241  18F11FF0   00000004    8        FF\t3F\t90\t68\t88\t1B\t10\t8C\r\n      3232  1FFFFFFF   00000004    8        00\t00\tFF\tFF\tFF\tFF\tFF\tFF\r\n      3223  0CF102A7   00000004    8        30\t75\tE0\t2E\t80\tFF\tFF\tFD\r\n      3223  0CF101A7   00000004    8        68\t00\t97\tCC\t00\t00\t39\tBB\r\n      3222  1FFFFFFF   00000004    8        00\t20\tFF\tFF\tFF\tFF\tFF\tFF\r\n      3212  1FFFFFFF   00000004    8        00\t00\tFF\tFF\tFF\tFF\tFF\tFF\r\n      3203  0CF102A7   00000004    8        30\t75\tE0\t2E\t80\tFF\tFF\tFD\r\n      3203  0CF101A7   00000004    8        68\t00\t97\tCC\t00\t16\t39\tBA\r\n      3202  1FFFFFFF   00000004    8        00\t00\tFF\tFF\tFF\tFF\tFF\tFF\r\n      3243  0C3C4D4A   00000004    8        BE\tFF\tFF\t7F\t18\tFF\tFF\t58\r\n      3243  0CF101A7   00000004    8        68\t00\t97\tCC\t00\t00\t39\tBC\r\n      3242  18F120F0   00000004    8        2B\t75\t60\tB1\tB0\t01\tFF\tFF\r\n      3241  18F11FF0   00000004    8        FF\t3F\t90\t68\t88\t1B\t10\t8C\r\n      3232  1FFFFFFF   00000004    8        00\t00\tFF\tFF\tFF\tFF\tFF\tFF\r\n      3223  0CF102A7   00000004    8        30\t75\tE0\t2E\t80\tFF\tFF\tFD\r\n      3223  0CF101A7   00000004    8        68\t00\t97\tCC\t00\t00\t39\tBB\r\n      3222  1FFFFFFF   00000004    8        00\t20\tFF\tFF\tFF\tFF\tFF\tFF\r\n      3212  1FFFFFFF   00000004    8        00\t00\tFF\tFF\tFF\tFF\tFF\tFF\r\n      3203  0CF102A7   00000004    8        30\t75\tE0\t2E\t80\tFF\tFF\tFD\r\n      3203  0CF101A7   00000004    8        68\t00\t97\tCC\t00\t16\t39\tBA\r\n      3244  0CF102A7   00000004    8        30\t75\tE0\t2E\t80\tFF\tFF\tFD\r\n      3243  0C3C4D4A   00000004    8        BE\tFF\tFF\t7F\t18\tFF\tFF\t58\r\n      3243  0CF101A7   00000004    8        68\t00\t97\tCC\t00\t00\t39\tBC\r\n      3242  18F120F0   00000004    8        2B\t75\t60\tB1\tB0\t01\tFF\tFF\r\n      3241  18F11FF0   00000004    8        FF\t3F\t90\t68\t88\t1B\t10\t8C\r\n      3232  1FFFFFFF   00000004    8        00\t00\tFF\tFF\tFF\tFF\tFF\tFF\r\n      3223  0CF102A7   00000004    8        30\t75\tE0\t2E\t80\tFF\tFF\tFD\r\n      3223  0CF101A7   00000004    8        68\t00\t97\tCC\t00\t00\t39\tBB\r\n      3222  1FFFFFFF   00000004    8        00\t20\tFF\tFF\tFF\tFF\tFF\tFF\r\n      3212  1FFFFFFF   00000004    8        00\t00\tFF\tFF\tFF\tFF\tFF\tFF\r\n      3203  0CF102A7   00000004    8        30\t75\tE0\t2E\t80\tFF\tFF\tFD\r\n      3244  0CF103A7   00000004    8        17\t1F\t08\t60\tB1\t1F\t08\t58\r\n      3244  0CF102A7   00000004    8        30\t75\tE0\t2E\t80\tFF\tFF\tFD\r\n      3243  0C3C4D4A   00000004    8        BE\tFF\tFF\t7F\t18\tFF\tFF\t58\r\n      3243  0CF101A7   00000004    8        68\t00\t97\tCC\t00\t00\t39\tBC\r\n      3242  18F120F0   00000004    8        2B\t75\t60\tB1\tB0\t01\tFF\tFF\r\n      3241  18F11FF0   00000004    8        FF\t3F\t90\t68\t88\t1B\t10\t8C\r\n      3232  1FFFFFFF   00000004    8        00\t00\tFF\tFF\tFF\tFF\tFF\tFF\r\n      3223  0CF102A7   00000004    8        30\t75\tE0\t2E\t80\tFF\tFF\tFD\r\n      3223  0CF101A7   00000004    8        68\t00\t97\tCC\t00\t00\t39\tBB\r\n      3222  1FFFFFFF   00000004    8        00\t20\tFF\tFF\tFF\tFF\tFF\tFF\r\n      3212  1FFFFFFF   00000004    8        00\t00\tFF\tFF\tFF\tFF\tFF\tFF\r\n      3245  0CF104A7   00000004    8        F0\t60\t22\tFC\tFF\tFF\tFF\t58\r\n      3244  0CF103A7   00000004    8        17\t1F\t08\t60\tB1\t1F\t08\t58\r\n      3244  0CF102A7   00000004    8        30\t75\tE0\t2E\t80\tFF\tFF\tFD\r\n      3243  0C3C4D4A   00000004    8        BE\tFF\tFF\t7F\t18\tFF\tFF\t58\r\n      3243  0CF101A7   00000004    8        68\t00\t97\tCC\t00\t00\t39\tBC\r\n      3242  18F120F0   00000004    8        2B\t75\t60\tB1\tB0\t01\tFF\tFF\r\n      3241  18F11FF0   00000004    8        FF\t3F\t90\t68\t88\t1B\t10\t8C\r\n      3232  1FFFFFFF   00000004    8        00\t00\tFF\tFF\tFF\tFF\tFF\tFF\r\n      3223  0CF102A7   00000004    8        30\t75\tE0\t2E\t80\tFF\tFF\tFD\r\n      3223  0CF101A7   00000004    8        68\t00\t97\tCC\t00\t00\t39\tBB\r\n      3222  1FFFFFFF   00000004    8        00\t20\tFF\tFF\tFF\tFF\tFF\tFF\r\n      3245  18F106A7   00000004    8        00\tF7\tFF\tFF\tFF\tFF\tFF\tB1\r\n      3245  0CF104A7   00000004    8        F0\t60\t22\tFC\tFF\tFF\tFF\t58\r\n      3244  0CF103A7   00000004    8        17\t1F\t08\t60\tB1\t1F\t08\t58\r\n      3244  0CF102A7   00000004    8        30\t75\tE0\t2E\t80\tFF\tFF\tFD\r\n      3243  0C3C4D4A   00000004    8        BE\tFF\tFF\t7F\t18\tFF\tFF\t58\r\n      3243  0CF101A7   00000004    8        68\t00\t97\tCC\t00\t00\t39\tBC\r\n      3242  18F120F0   00000004    8        2B\t75\t60\tB1\tB0\t01\tFF\tFF\r\n      3241  18F11FF0   00000004    8        FF\t3F\t90\t68\t88\t1B\t10\t8C\r\n      3232  1FFFFFFF   00000004    8        00\t00\tFF\tFF\tFF\tFF\tFF\tFF\r\n      3223  0CF102A7   00000004    8        30\t75\tE0\t2E\t80\tFF\tFF\tFD\r\n      3223  0CF101A7   00000004    8        68\t00\t97\tCC\t00\t00\t39\tBB\r\n      3246  18F121F0   00000004    8        09\t33\t00\t00\tFF\tFF\tB0\t01\r\n      3245  18F106A7   00000004    8        00\tF7\tFF\tFF\tFF\tFF\tFF\tB1\r\n      3245  0CF104A7   00000004    8        F0\t60\t22\tFC\tFF\tFF\tFF\t58\r\n      3244  0CF103A7   00000004    8        17\t1F\t08\t60\tB1\t1F\t08\t58\r\n      3244  0CF102A7   00000004    8        30\t75\tE0\t2E\t80\tFF\tFF\tFD\r\n      3243  0C3C4D4A   00000004    8        BE\tFF\tFF\t7F\t18\tFF\tFF\t58\r\n      3243  0CF101A7   00000004    8        68\t00\t97\tCC\t00\t00\t39\tBC\r\n      3242  18F120F0   00000004    8        2B\t75\t60\tB1\tB0\t01\tFF\tFF\r\n      3241  18F11FF0   00000004    8        FF\t3F\t90\t68\t88\t1B\t10\t8C\r\n      3232  1FFFFFFF   00000004    8        00\t00\tFF\tFF\tFF\tFF\tFF\tFF\r\n      3223  0CF102A7   00000004    8        30\t75\tE0\t2E\t80\tFF\tFF\tFD\r\n      3247  1FFFFFFF   00000004    8        00\t00\tFF\tFF\tFF\tFF\tFF\tFF\r\n      3246  18F121F0   00000004    8        09\t33\t00\t00\tFF\tFF\tB0\t01\r\n      3245  18F106A7   00000004    8        00\tF7\tFF\tFF\tFF\tFF\tFF\tB1\r\n      3245  0CF104A7   00000004    8        F0\t60\t22\tFC\tFF\tFF\tFF\t58\r\n      3244  0CF103A7   00000004    8        17\t1F\t08\t60\tB1\t1F\t08\t58\r\n      3244  0CF102A7   00000004    8        30\t75\tE0\t2E\t80\tFF\tFF\tFD\r\n      3243  0C3C4D4A   00000004    8        BE\tFF\tFF\t7F\t18\tFF\tFF\t58\r\n      3243  0CF101A7   00000004    8        68\t00\t97\tCC\t00\t00\t39\tBC\r\n      3242  18F120F0   00000004    8        2B\t75\t60\tB1\tB0\t01\tFF\tFF\r\n      3241  18F11FF0   00000004    8        FF\t3F\t90\t68\t88\t1B\t10\t8C\r\n      3232  1FFFFFFF   00000004    8        00\t00\tFF\tFF\tFF\tFF\tFF\tFF\r\n      3252  1FFFFFFF   00000004    8        00\t00\tFF\tFF\tFF\tFF\tFF\tFF\r\n      3247  1FFFFFFF   00000004    8        00\t00\tFF\tFF\tFF\tFF\tFF\tFF\r\n      3246  18F121F0   00000004    8        09\t33\t00\t00\tFF\tFF\tB0\t01\r\n      3245  18F106A7   00000004    8        00\tF7\tFF\tFF\tFF\tFF\tFF\tB1\r\n      3245  0CF104A7   00000004    8        F0\t60\t22\tFC\tFF\tFF\tFF\t58\r\n      3244  0CF103A7   00000004    8        17\t1F\t08\t60\tB1\t1F\t08\t58\r\n      3244  0CF102A7   00000004    8        30\t75\tE0\t2E\t80\tFF\tFF\tFD\r\n      3243  0C3C4D4A   00000004    8        BE\tFF\tFF\t7F\t18\tFF\tFF\t58\r\n      3243  0CF101A7   00000004    8        68\t00\t97\tCC\t00\t00\t39\tBC\r\n      3242  18F120F0   00000004    8        2B\t75\t60\tB1\tB0\t01\tFF\tFF\r\n      3241  18F11FF0   00000004    8        FF\t3F\t90\t68\t88\t1B\t10\t8C\r\n      3262  1FFFFFFF   00000004    8        00\t00\tFF\tFF\tFF\tFF\tFF\tFF\r\n      3252  1FFFFFFF   00000004    8        00\t00\tFF\tFF\tFF\tFF\tFF\tFF\r\n      3247  1FFFFFFF   00000004    8        00\t00\tFF\tFF\tFF\tFF\tFF\tFF\r\n      3246  18F121F0   00000004    8        09\t33\t00\t00\tFF\tFF\tB0\t01\r\n      3245  18F106A7   00000004    8        00\tF7\tFF\tFF\tFF\tFF\tFF\tB1\r\n      3245  0CF104A7   00000004    8        F0\t60\t22\tFC\tFF\tFF\tFF\t58\r\n      3244  0CF103A7   00000004    8        17\t1F\t08\t60\tB1\t1F\t08\t58\r\n      3244  0CF102A7   00000004    8        30\t75\tE0\t2E\t80\tFF\tFF\tFD\r\n      3243  0C3C4D4A   00000004    8        BE\tFF\tFF\t7F\t18\tFF\tFF\t58\r\n      3243  0CF101A7   00000004    8        68\t00\t97\tCC\t00\t00\t39\tBC\r\n      3242  18F120F0   00000004    8        2B\t75\t60\tB1\tB0\t01\tFF\tFF\r\n      3263  0CF101A7   00000004    8        68\t00\t97\tCC\t00\t19\t39\tBD\r\n      3262  1FFFFFFF   00000004    8        00\t00\tFF\tFF\tFF\tFF\tFF\tFF\r\n      3252  1FFFFFFF   00000004    8        00\t00\tFF\tFF\tFF\tFF\tFF\tFF\r\n      3247  1FFFFFFF   00000004    8        00\t00\tFF\tFF\tFF\tFF\tFF\tFF\r\n      3246  18F121F0   00000004    8        09\t33\t00\t00\tFF\tFF\tB0\t01\r\n      3245  18F106A7   00000004    8        00\tF7\tFF\tFF\tFF\tFF\tFF\tB1\r\n      3245  0CF104A7   00000004    8        F0\t60\t22\tFC\tFF\tFF\tFF\t58\r\n      3244  0CF103A7   00000004    8        17\t1F\t08\t60\tB1\t1F\t08\t58\r\n      3244  0CF102A7   00000004    8        30\t75\tE0\t2E\t80\tFF\tFF\tFD\r\n      3243  0C3C4D4A   00000004    8        BE\tFF\tFF\t7F\t18\tFF\tFF\t58\r\n      3243  0CF101A7   00000004    8        68\t00\t97\tCC\t00\t00\t39\tBC\r\n      3263  0CF102A7   00000004    8        30\t75\tE0\t2E\t80\tFF\tFF\tFD\r\n      3263  0CF101A7   00000004    8        68\t00\t97\tCC\t00\t19\t39\tBD\r\n      3262  1FFFFFFF   00000004    8        00\t00\tFF\tFF\tFF\tFF\tFF\tFF\r\n      3252  1FFFFFFF   00000004    8        00\t00\tFF\tFF\tFF\tFF\tFF\tFF\r\n      3247  
